vi "Update Preview Graph.vi"(9 "Plot Visible Array":refnum<vi>, 10 "Settings In":T1, 11 "Graph Preview Ref":refnum<vi>) -> ()   [LabVIEW 2020, in "Sequencer with Output Values.lvlib" / "Sequencer with Output Values.lvclass"]
uses:
  Sequencer with Output Values.lvclass
  Params.ctl
  Step Settings.ctl
  Global Strings.vi
panel:
  out "Waveform Graph":waveform(dbl)[](graph)
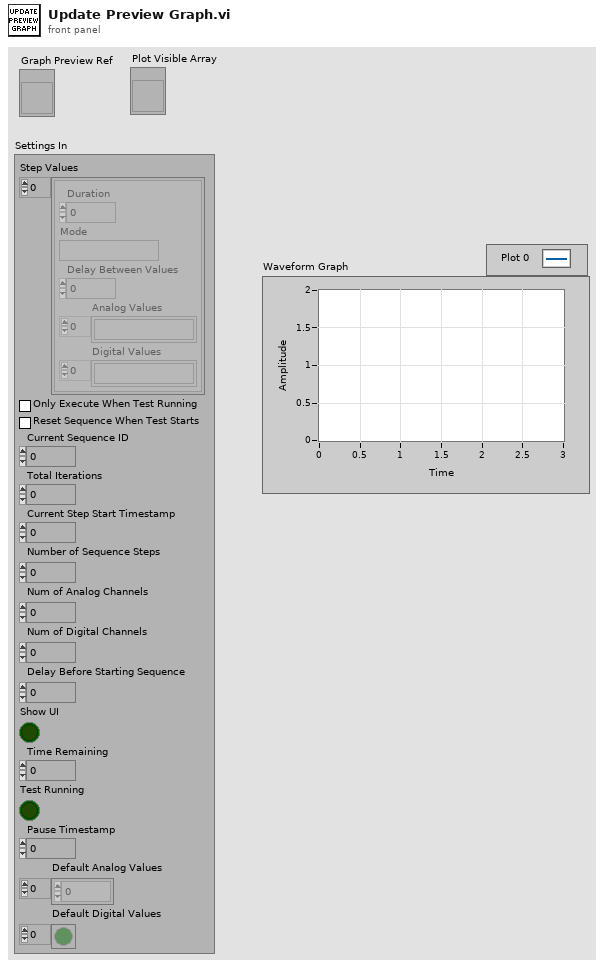
[diagram p1: front panel]
types:
  T1 = typedef "Sequencer with Output Values.lvlib/Sequencer with Output Values.lvclass/Params.ctl" = cluster{"Step Values":T2[], "Only Execute When Test Running":bool, "Reset Sequence When Test Starts":bool, "Current Sequence ID":u32, "Total Iterations":u32, "Current Step Start Timestamp":dbl, "Number of Sequence Steps":i32, "Num of Analog Channels":i32, "Num of Digital Channels":i32, "Delay Before Starting Sequence":dbl, "Show UI":bool, "Time Remaining":dbl, "Test Running":bool, "Pause Timestamp":dbl, "Default Analog Values":dbl[], "Default Digital Values":bool[]}
  T2 = typedef "Sequencer with Output Values.lvlib/Sequencer with Output Values.lvclass/Step Settings.ctl" = cluster{"Duration":dbl, "Mode":string, "Delay Between Values":dbl, "Analog Values":string[], "Digital Values":string[]}
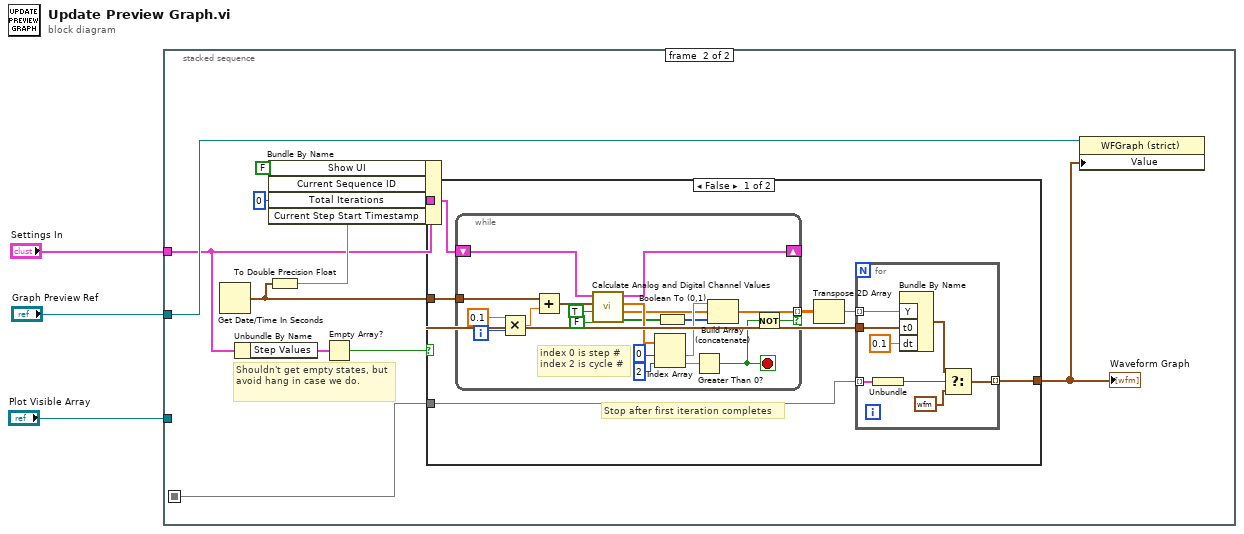
[diagram p0: block diagram]
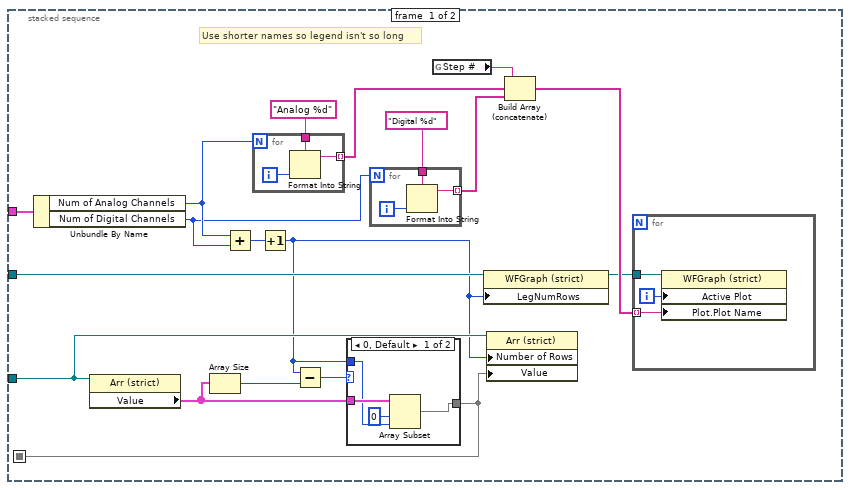
[diagram p2: hidden frame]
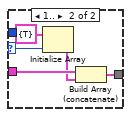
[diagram p3: hidden frame]
diagram:
  n1 = stacked-sequence {
    seq-local: [w4 _] -> [_ w40]
    tunnel: "Settings In" -> [w21 w44]
    tunnel: "Graph Preview Ref" -> [w20 w47]
    tunnel: "Plot Visible Array" -> [w13 _]
    frame #0 {
      # "Use shorter names so legend isn't so long"
      n2 = Unbundle By Name(w21) -> ("Num of Analog Channels"=w19:i32, "Num of Digital Channels"=w18:i32)
      n3 = property class="Arr (strict)"(reference=w13) -> ("Value"=w6:cluster{"Boolean 2":bool}[])  [unwired: 1 in, 2 out]
      n4 = Array Size(array=w6) -> (size(s)=w8:i32)
      n5 = Add(x=w19, y=w18) -> (x+y=w17:i32)
      n6 = for {
        N: w19 -> [_]
        tunnel: "Analog %d" -> [w38]
        tunnel: [w37] -> w10 mode=indexing
        i -> [w39]
        n7 = Format Into String(format string=w38, w39) -> (resulting string=w37:string)  [unwired: 2 in, 1 out]
      }
      n8 = Increment(x=w17) -> (x+1=w5:i32)
      n9 = Subtract(x=w5, y=w8) -> (x-y=w7:i32)
      n10 = case shown="0, Default" w7 {
        selector: w7 -> [_ w30]
        tunnel: w6 -> [w25 w28]
        tunnel: [w22 w26] -> w4
        tunnel: w5 -> [w23 _]
        frame 0, Default {
          n11 = Array Subset(array=w25, index=0, length=w23) -> (w22:cluster{"Boolean 2":bool}[])
        }
        frame 1.. {
          n12 = Initialize Array(cluster{"Boolean 2":bool} {"Boolean 2"=TRUE} ("Cluster"), w30) -> (w27:cluster{"Boolean 2":bool}[])
          n13 = Build Array (concatenate)(w28, w27) -> (w26:cluster{"Boolean 2":bool}[])
        }
      }
      n14 = for {
        N: w18 -> [_]
        tunnel: "Digital %d" -> [w35]
        tunnel: [w34] -> w9 mode=indexing
        i -> [w36]
        n15 = Format Into String(format string=w35, w36) -> (resulting string=w34:string)  [unwired: 2 in, 1 out]
      }
      n16 = global read "Global Strings.vi" "Step #"() -> (w15:string)
      n17 = property class="WFGraph (strict)"(reference=w20, "LegNumRows"=w5) -> (reference out=w14:refnum<vi>)  [unwired: 1 in, 1 out]
      n18 = property class="Arr (strict)"(reference=w13, "Number of Rows"=w5, "Value"=w4) -> ()  [unwired: 1 in, 2 out]
      n19 = Build Array (concatenate)(w15, w10, w9) -> (w16:string[])
      n20 = for {
        tunnel: w14 -> [w33]
        tunnel: w16 -> [w31] mode=indexing
        i -> [w32]
        n21 = property class="WFGraph (strict)"(reference=w33, "Active Plot"=w32, "Plot.Plot Name"=w31) -> ()  [unwired: 1 in, 2 out]
      }
    }
    frame #1 {
      w48 = u32 0 ("Total Iterations")
      # "Shouldn't get empty states, but avoid hang in case we do."
      n22 = Get Date/Time In Seconds() -> (seconds since 1Jan1904=w46:timestamp)
      n23 = Unbundle By Name(w44) -> ("Step Values"=w43:T2[])
      n24 = To Double Precision Float(number=w46) -> (double precision float=w49:dbl)
      n25 = Bundle By Name(cluster=w44, "Show UI"=FALSE, "Current Sequence ID"=w48, "Total Iterations"=w48, "Current Step Start Timestamp"=w49) -> (w50:T1)
      n26 = Empty Array?(array=w43) -> (empty?=w42:bool)
      n27 = case shown="False" w42 {
        tunnel: w50 -> [w56 _]
        tunnel: w46 -> [w54 _]
        tunnel: [w51 _] -> w45
        tunnel: w40 -> [w52 _]
        frame False {
          # "Stop after first iteration completes"
          n28 = while {
            shift-right: [w70] -> _
            shift-left: w56 -> [w72]
            tunnel: w54 -> [w82]
            tunnel: [w75] -> w55 mode=indexing if=w73
            i -> [w84]
            stop <- w74 stop-if-true
            # "index 0 is step #\nindex 2 is cycle #"
            n29 = Multiply(x=0.1, y=w84) -> (x*y=w81:dbl)
            n30 = Add(x=w82, y=w81) -> (x+y=w71:timestamp)
            n31 = call "Calculate Analog and Digital Channel Values.vi"("Use Default Values"=FALSE, "Execute Sequence"=TRUE, "current time"=w71, "Settings in"=w72) -> ("Digital Values to Write"=w67:bool[], "Analog Values to Write"=w68:dbl[], "Sequence State Channels to Write"=w69:dbl[], "Settings out"=w70:T1)  [unwired: 4 in]
            n32 = Index Array(array=w69, index #1=0 ("index"), index #2=2 ("index")) -> (element #1=w78:dbl, element #2=w79:dbl)
            n33 = Boolean To (0,1)(Boolean=w67) -> (0, 1=w76:i16[])
            n34 = Greater Than 0?(x=w79) -> (x > 0?=w74:bool)
            n35 = Build Array (concatenate)(w78, w68, w76) -> (w75:dbl[])
            n36 = Not(x=w74) -> (.not. x?=w73:bool)
          }
          n37 = Transpose 2D Array(2D array=w55) -> (transposed array=w53:dbl[][])
          n38 = for {
            tunnel: w53 -> [w64] mode=indexing
            tunnel: w54 -> [w63]
            tunnel: w52 -> [w61] mode=indexing
            tunnel: [w58] -> w51 mode=indexing
            n39 = Unbundle(w61) -> ("Boolean 2"=w60:bool)
            n40 = Bundle By Name("Y"=w64, "t0"=w63, "dt"=0.1) -> (w59:waveform(dbl))  [unwired: 1 in]
            n41 = Select(t=w59, s=w60, f=waveform(dbl) {"t0"=timestamp(0 s since 1904-01-01), "dt"=1.0, "Y"=[]}) -> (s? t:f=w58:waveform(dbl))
          }
        }
        frame True {
        }
      }
      "Waveform Graph" <- w45
      n42 = property class="WFGraph (strict)"(reference=w47, "Value"=w45) -> ()  [unwired: 1 in, 2 out]
    }
  }
